vi "DSB Modulation.vi"() -> ()   [LabVIEW 2013]
uses:
  <vilib>/sound2/lvsound2.llb/Sound File Info (path).vi
  <vilib>/sound2/lvsound2.llb/Sound File Read Open.vi
  <vilib>/sound2/lvsound2.llb/Sound File Read (DBL).vi
  <vilib>/Waveform/WDTOps.llb/WDT Get Waveform Subset DBL.vi
  <vilib>/express/express analysis/Spectral/Block/exnSpectralBlock spectral measurements power poly.vi
  <vilib>/express/express analysis/Spectral/Block/exnSpectralBlock spectral measurements power DDT.vi
  <vilib>/express/express analysis/Spectral/Block/exnSpectralBlock spectral measurements RMS poly.vi
  <vilib>/express/express analysis/Spectral/Block/exnSpectralBlock spectral measurements RMS DDT.vi
  <vilib>/express/express analysis/Spectral/XNode/ExpressSpectralMeasurementsBlockNode.xnode
panel:
  out "After BPF":dynamicdata(graph)
  in  "Modulated Signal Source":enum32{"Single Tone", "From File"}(tab)
  in  "ST Frequency":dbl=2000.0 caption="Frequency"
  in  "ST Amplitude":dbl=1.0 caption="Amplitude"
  in  "Resample Rate":dbl=1000000.0 format="%#_6f"
  in  "Duration":dbl=44100.0
  in  "WAV Path":path caption="Path"
  out "DSB Squared":dynamicdata(graph)
  out "Estimated Freq.":dbl caption="Amplitude" format="%#_9g"
  in  "WAV Sample Rate":dbl=44100.0 caption="dt"
  in  "LPF Cut-Off":dbl=50000.0 caption="Lower Cut-Off"
  in  "SNR (dB)":dbl(slide)=30.0 caption="Standard deviation" scale=-20.0..30.0
  out "Comparision":dynamicdata(graph)
  out "Baseband":dynamicdata(graph)
  out "DSB FFT":dynamicdata(graph)
  out "DSB Wave":dynamicdata(graph)
  in  "Carrier Amp.":dbl=1.0 caption="Amplitude"
  in  "stop":bool
  in  "Frequency Offset":dbl(slide) scale=-1000.0..1000.0
  in  "Carrier Freq.":dbl=100000.0 caption="Frequency"
  # "DSB Modulation"
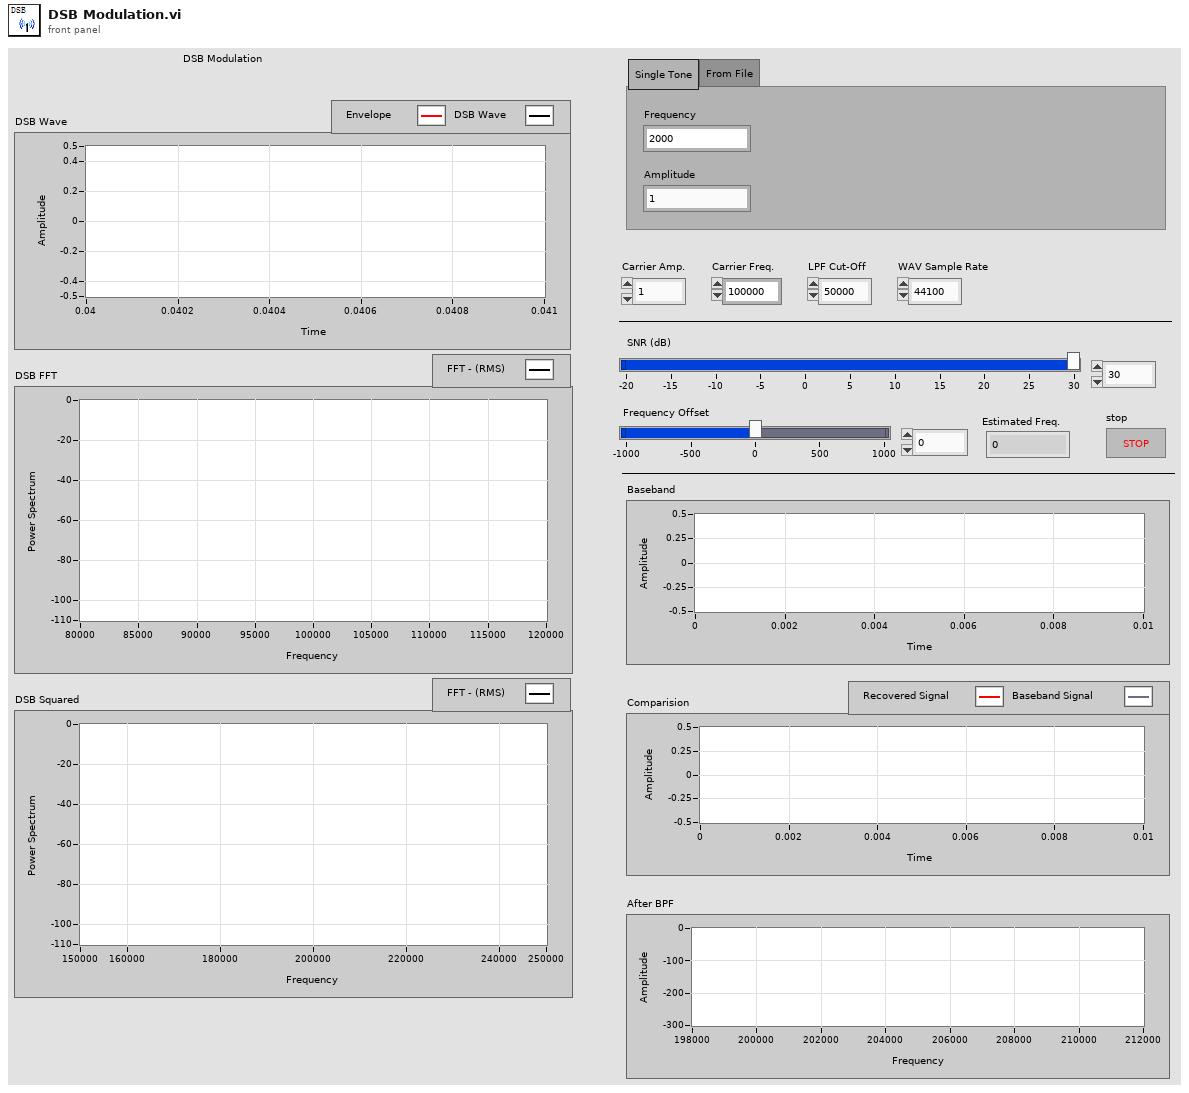
[diagram p1: front panel]
types:
  T1 = typedef "Sound File Refnum.ctl" = refnum<file>
  T2 = cluster{"averaging mode":u16, "weighting mode":u16, "number of averages":u32}
  T3 = cluster{"dB On (F)":bool, "unwrap phase (F)":bool, "convert to degree (F)":bool}
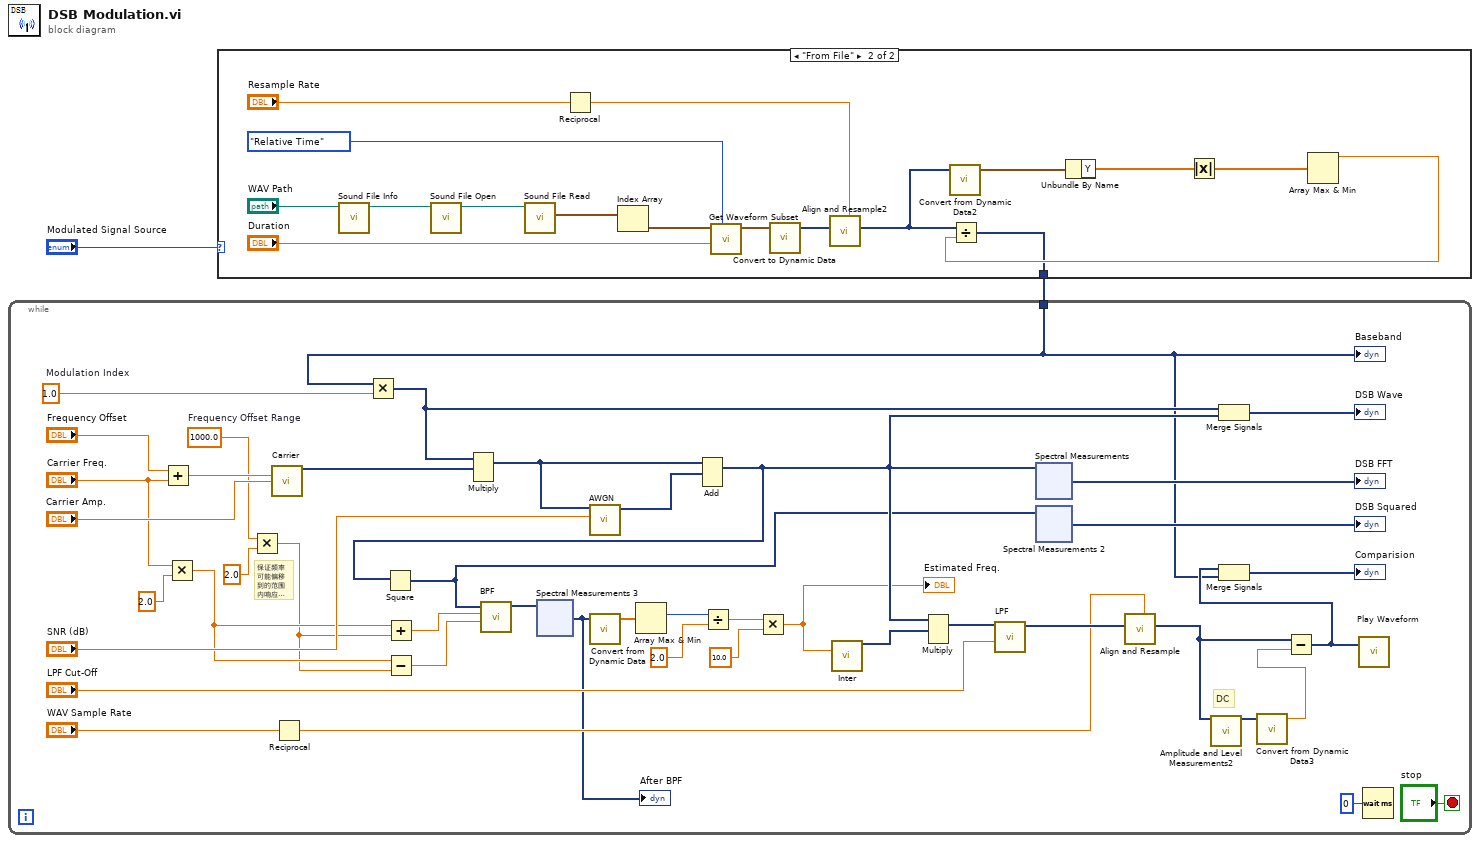
[diagram p0: block diagram]
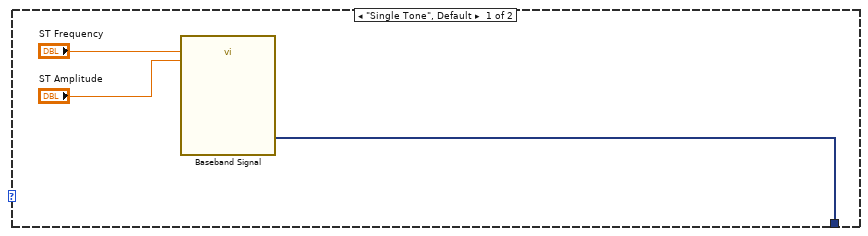
[diagram p2: hidden frame]
diagram:
  n1 = case shown="\"From File\"" "Modulated Signal Source" {
    tunnel: [w3 w7] -> w1
    frame "Single Tone", Default {
      n2 = call "Baseband Signal"("Frequency"="ST Frequency", "Amplitude"="ST Amplitude") -> ("Sine"=w3:dynamicdata)  [unwired: 12 in, 1 out]
    }
    frame "From File" {
      n3 = call-poly <vilib>:"Sound File Info.vi"("path"="WAV Path") -> ("path out"=w20:path)  [unwired: 7 in, 3 out]
      n4 = call-poly <vilib>:"Sound File Open.vi"("path"=w20) -> ("sound file refnum"=w22:T1)  [unwired: 9 in, 1 out]
      n5 = call-poly <vilib>:"Sound File Read.vi"("sound file refnum"=w22) -> ("data"=w17:waveform(dbl)[])  [unwired: 6 in, 4 out]
      n6 = Reciprocal(x="Resample Rate") -> (1/x=w13:dbl)
      n7 = Index Array(array=w17) -> (element=w18:waveform(dbl))  [unwired: 1 in]
      n8 = call-poly <vilib>:"Get Waveform Subset.vi"("start/duration format"=enum16{"Relative Time"}."Relative Time", "duration"="Duration", "waveform in"=w18) -> ("waveform out"=w12:waveform(dbl))  [unwired: 3 in, 3 out]
      n9 = call "Convert to Dynamic Data"("Waveform"=w12) -> ("Dynamic Data Type"=w6:dynamicdata)  [unwired: 3 in]
      n10 = call "Align and Resample2"("dt"=w13, "Signals"=w6) -> ("Resampled Signals"=w8:dynamicdata)  [unwired: 7 in, 2 out]
      n11 = call "Convert from Dynamic Data2"("Dynamic Data Type"=w8) -> ("Waveform"=w15:waveform(dbl))  [unwired: 3 in]
      n12 = Unbundle By Name(w15) -> ("Y"=w9:dbl[])
      n13 = Absolute Value(x=w9) -> (abs(x)=w11:dbl[])
      n14 = Array Max & Min(array=w11) -> (max value=w10:dbl)  [unwired: 3 out]
      n15 = Divide(x=w8, y=w10) -> (x/y=w7:dynamicdata)
    }
  }
  n16 = while {
    tunnel: w1 -> [w29]
    stop <- "stop" stop-if-true
    w23 = 1000.0  # Frequency Offset Range
    w60 = 1.0  # Modulation Index
    # "保证频率可能偏移到的范围内响应是平的"
    # "DC"
    n17 = Add(x="Frequency Offset", y="Carrier Freq.") -> (x+y=w59:dbl)
    n18 = Multiply(x="Carrier Freq.", y=2.0) -> (x*y=w33:dbl)
    n19 = Multiply(x=w23, y=2.0) -> (x*y=w24:dbl)
    n20 = call "Carrier"("Frequency"=w59, "Amplitude"="Carrier Amp.") -> ("Sine"=w56:dynamicdata)  [unwired: 12 in, 1 out]
    n21 = Reciprocal(x="WAV Sample Rate") -> (1/x=w49:dbl)
    n22 = Multiply(x=w29, y=w60) -> (x*y=w55:dynamicdata)
    n23 = Add(x=w33, y=w24) -> (x+y=w31:dbl)
    n24 = Subtract(x=w33, y=w24) -> (x-y=w30:dbl)
    n25 = Multiply(1:w56, 2:w55) -> (0:w54:dynamicdata)  [unwired: 1 in, 1 out]
    n26 = call "AWGN.vi"("SNR (dB)"="SNR (dB)", "Dynamic Data"=w54) -> ("DC with Gaussian Noise"=w53:dynamicdata)  [unwired: 9 in]
    n27 = Add(1:w53, 2:w54) -> (0:w41:dynamicdata)  [unwired: 1 in, 1 out]
    n28 = Square(x=w41) -> (x^2=w26:dynamicdata)
    n29 = call "BPF"("Lower Cut-Off"=w30, "Upper Cut-Off"=w31, "Signal"=w26) -> ("Filtered Signal"=w27:dynamicdata)  [unwired: 7 in, 1 out]
    n30 = xnode ("Spectral Measurements 3")("Signals"=w27) -> ("Power Spectrum"=w28:dynamicdata)  [unwired: 1 in, 1 out]
    "After BPF" <- w28
    n31 = call "Convert from Dynamic Data"("Dynamic Data Type"=w28) -> ("Array"=w40:dbl[])  [unwired: 3 in]
    n32 = Array Max & Min(array=w40) -> (max index (indices)=w37:i32)  [unwired: 3 out]
    n33 = Divide(x=w37, y=2.0) -> (x/y=w38:dbl)
    n34 = Multiply(x=w38, y=10.0) -> (x*y=w39:dbl)
    "Estimated Freq." <- w39
    n35 = call "Inter"("Frequency"=w39) -> ("Sine"=w43:dynamicdata)  [unwired: 13 in, 1 out]
    n36 = Multiply(1:w43, 2:w41) -> (0:w44:dynamicdata)  [unwired: 1 in, 1 out]
    n37 = call "LPF"("Lower Cut-Off"="LPF Cut-Off", "Signal"=w44) -> ("Filtered Signal"=w51:dynamicdata)  [unwired: 8 in, 1 out]
    n38 = xnode ("Spectral Measurements")("Signals"=w41) -> ("FFT - (RMS)"=→"DSB FFT":dynamicdata)  [unwired: 1 in, 2 out]
    n39 = xnode ("Spectral Measurements 2")("Signals"=w26) -> ("FFT - (RMS)"=→"DSB Squared":dynamicdata)  [unwired: 1 in, 2 out]
    n40 = call "Align and Resample"("dt"=w49, "Signals"=w51) -> ("Resampled Signals"=w63:dynamicdata)  [unwired: 7 in, 2 out]
    n41 = call "Amplitude and Level Measurements2"("Signals"=w63) -> ("Mean (DC)"=w65:dynamicdata)  [unwired: 13 in, 1 out]
    n42 = Merge Signals(w55, w41) -> (→"DSB Wave":dynamicdata)
    n43 = call "Convert from Dynamic Data3"("Dynamic Data Type"=w65) -> ("Scalar"=w62:dbl)  [unwired: 3 in]
    n44 = Subtract(x=w63, y=w62) -> (x-y=w47:dynamicdata)
    n45 = Merge Signals(w47, w29) -> (→"Comparision":dynamicdata)
    n46 = call "Play Waveform"("Data"=w47) -> ()  [unwired: 18 in, 1 out]
    n47 = Wait (ms)(milliseconds to wait=u32 0) -> ()  [unwired: 1 out]
    "Baseband" <- w29
  }
